vi "GOOP_OCREvaluation.vi"(10 "OcrText":string="DatCfg", 11 "Viname":string="MtDataConfiguration") -> (3 "Match":bool)   [LabVIEW 2020]
panel:
  out "Boolean":bool
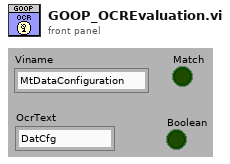
[diagram p1: front panel]
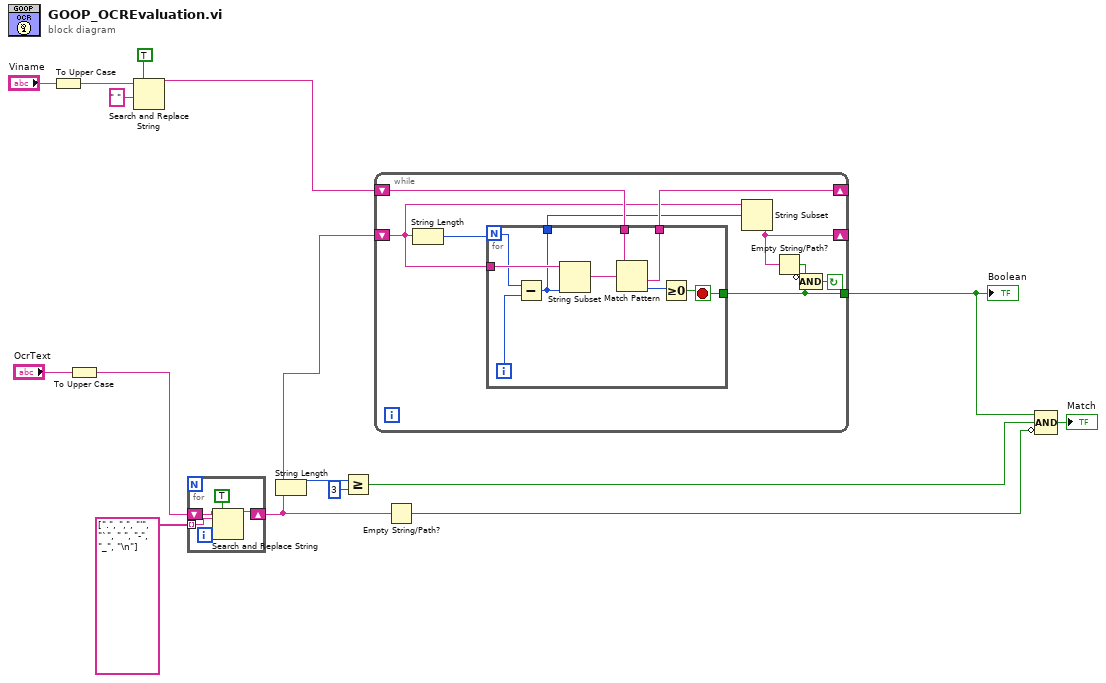
[diagram p0: block diagram]
diagram:
  n1 = To Upper Case(1:"Viname") -> (0:w15:string)
  n2 = To Upper Case(1:"OcrText") -> (0:w1:string)
  n3 = Search and Replace String(replace all?=TRUE ("replace all? (F)"), input string=w15, search string=" ") -> (result string=w4:string)  [unwired: 5 in, 3 out]
  n4 = for {
    shift-right: [w18] -> w2
    shift-left: w1 -> [w19]
    tunnel: string[] [".", ",", "'", "`", " ", "-", "_", "\n"] -> [w16] mode=indexing
    n5 = Search and Replace String(replace all?=TRUE ("replace all? (F)"), input string=w19, search string=w16) -> (result string=w18:string)  [unwired: 5 in, 3 out]
  }
  n6 = String Length(string=w2) -> (length=w10:i32)
  n7 = Greater Or Equal?(x=w10, y=3) -> (x >= y?=w8:bool)
  n8 = while {
    shift-right: [w24] -> _
    shift-left: w2 -> [w25]
    shift-right: [w26] -> _
    shift-left: w4 -> [w27]
    tunnel: [w21] -> w3
    stop <- w22 continue-if-true
    n9 = String Length(string=w25) -> (length=w28:i32)
    n10 = for {
      N: w28 -> [w36]
      tunnel: w25 -> [w37]
      tunnel: w27 -> [w34]
      tunnel: [w31] -> w26
      tunnel: [w30] -> w20
      tunnel: [w29] -> w21
      i -> [w35]
      stop <- w29 stop-if-true
      n11 = Subtract(x=w36, y=w35) -> (x-y=w30:i32)
      n12 = String Subset(string=w37, length (rest)=w30) -> (substring=w32:string)  [unwired: 1 in]
      n13 = Match Pattern(string=w34, regular expression=w32) -> (after substring=w31:string, offset past match=w33:i32)  [unwired: 1 in, 2 out]
      n14 = Greater Or Equal To 0?(x=w33) -> (x >= 0?=w29:bool)
    }
    n15 = String Subset(string=w25, offset (0)=w20) -> (substring=w24:string)  [unwired: 1 in]
    n16 = Empty String/Path?(string/path=w24) -> (empty?=w23:bool)
    n17 = Compound Arithmetic op=AND(invert w23, w21) -> (w22:bool)
  }
  "Boolean" <- w3
  n18 = Empty String/Path?(string/path=w2) -> (empty?=w12:bool)
  n19 = Compound Arithmetic op=AND(w3, w8, invert w12) -> (→"Match":bool)
